vi "HB_ImaqSnap.vi"() -> ()   [LabVIEW 2009]
doc: "The HL Snap VI acquires an image and displays the image in an image control using the high-level acquisition VIs. A snap is appropriate for low-speed or single-capture applications where ease of programming is essential.\n\nIMAQ Init initializes the device. IMAQ Create creates an image buffer. IMAQ Snap acquires an image into the buffer, and an image control displays the image on the front panel. IMAQ Close releases resources associated with the acquisition, and the IMAQ Dispose frees the image buffer. Use this sequence to ensure that the image control displays the image before the memory is disposed."
uses:
  lib.lib/HGF_LVC/HGF_IMAQ/HGF_IMAQFactory/HGF_IMAQFactory.lvclass
  lib.lib/HGF_LVC/HGF_IMAQ/HGF_IMAQDevice/HGF_IMAQDevice.lvclass
  lib.lib/HGF_LVC/HGF_BaseClasses/HGF_Factory/HGF_Factory.lvclass
  lib.lib/HGF_LVC/HGF_DeviceBaseClasses/HGF_DeviceBase/HGF_DeviceBase.lvclass
  lib.lib/HGF_LVC/HGF_Auxiliary/HGF_Auxiliary.lvlib
panel:
  out "iteration":i32
  out "Image":T1(plugin-control)
  in  "interval / ms":u32=100
  in  "stop":bool
  in  "Image Type":T2 items=["Grayscale (U8)", "Grayscale (I16)", "Grayscale (SGL)", "Complex (CSG)", "RGB (U32)", "HSL (U32)", "RGB (U64)", "Grayscale (U16)"]
  in  "cameraName":string="cam0"
  in  "imaqClassName":string="HGF_ImaqDx"
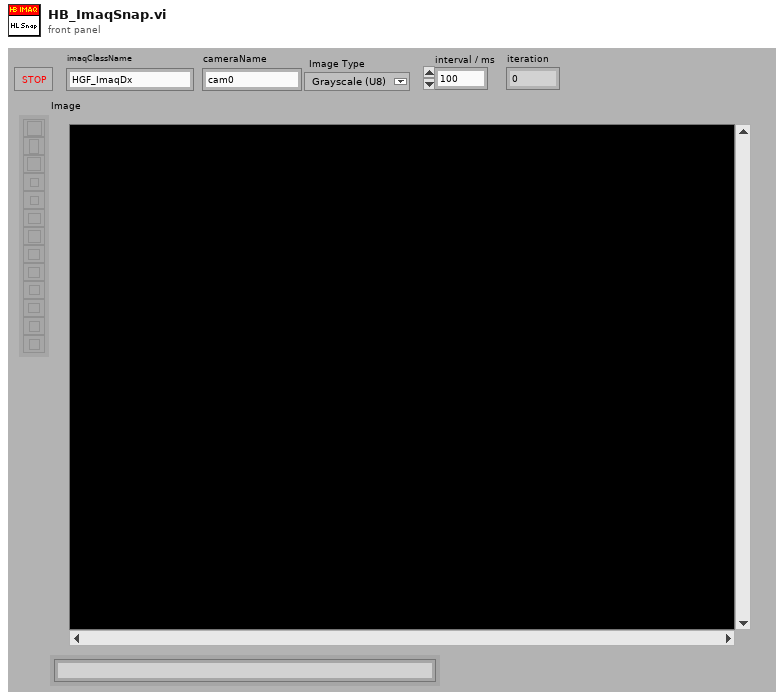
[diagram p1: front panel]
types:
  T1 = typedef "IMAQ Image.ctl" = refnum<image>
  T2 = typedef "Image Type" = u32
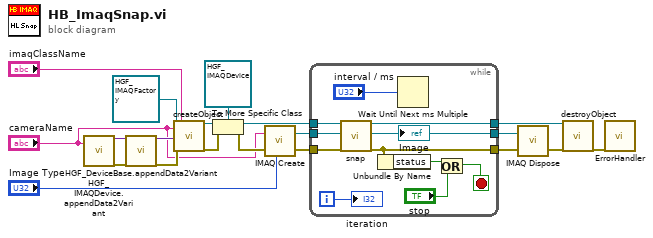
[diagram p0: block diagram]
diagram:
  n1 = call "HGF_IMAQDevice.appendData2Variant.vi"("cameraName"="cameraName") -> ("dup initData"=w20:variant, "error out"=w19:errorcluster)  [unwired: 5 in, 12 out]
  n2 = call "HGF_DeviceBase.appendData2Variant.vi"("initData"=w20, "error in (no error)"=w19) -> ("dup initData"=w17:variant, "error out"=w18:errorcluster)  [unwired: 16 out]
  n3 = call "createObject.vi"("HGF_Factory"=refnum<class "HGF_IMAQFactory.lvclass"> refnum ("HGF_IMAQ.lvlib:HGF_IMAQFactory.lvclass"), "objectName"="cameraName", "initializationData"=w17, "error in (no error)"=w18, "className"="imaqClassName") -> ("HGF_Object"=w14:refnum<class "HGF_Factory.lvclass">, "error out"=w13:errorcluster)  [unwired: 13 out]
  n4 = To More Specific Class(target class=refnum<class "HGF_IMAQDevice.lvclass"> refnum ("HGF_DeviceBaseClasses.lvlib:HGF_IMAQDevice.lvclass"), reference=w14, error in=w13) -> (specific class reference=w11:refnum<class "HGF_IMAQDevice.lvclass">, error out=w10:errorcluster)
  n5 = call "IMAQ Create"("Image Name"="cameraName", "Image Type"="Image Type", "error in (no error)"=w10) -> ("New Image"=w8:T1, "error out"=w9:errorcluster)  [unwired: 1 in, 1 out]
  n6 = while {
    tunnel: w11 -> [w31]
    tunnel: w9 -> [w30]
    tunnel: w8 -> [w29]
    tunnel: [w22] -> w5
    tunnel: [w27] -> w4
    tunnel: [w28] -> w2
    i -> [w21]
    stop <- w24 stop-if-true
    n7 = call "snap.vi"("HGF_IMAQDevice"=w31, "Image In"=w29, "error in (no error)"=w30) -> ("dup HGF_IMAQDevice"=w28:refnum<class "HGF_IMAQDevice.lvclass">, "Image Out"=w22:T1, "error out"=w27:errorcluster)  [unwired: 14 out]
    "Image" <- w22
    n8 = Unbundle By Name(w27) -> ("status"=w26:bool)
    n9 = Wait Until Next ms Multiple(millisecond multiple="interval / ms") -> ()  [unwired: 1 out]
    n10 = Or(x=w26, y="stop") -> (x .or. y?=w24:bool)
    "iteration" <- w21
  }
  n11 = call "IMAQ Dispose"("Image"=w5, "error in (no error)"=w4) -> ("error out"=w3:errorcluster)  [unwired: 1 in, 3 out]
  n12 = call "destroyObject.vi"("HGF_Factory"=w2, "error in (no error)"=w3) -> ("error out"=w1:errorcluster)  [unwired: 17 out]
  n13 = call "ErrorHandler.vi"("error in (no error)"=w1) -> ()  [unwired: 6 in, 13 out]
